vi "Opgave 9 Coolprop.vi"(10 "Temperatur":dbl, 11 "Tryk":dbl) -> (2 "Error Out":errorcluster, 3 "Entropy [kJ/kg-K]":dbl)   [LabVIEW 2019]
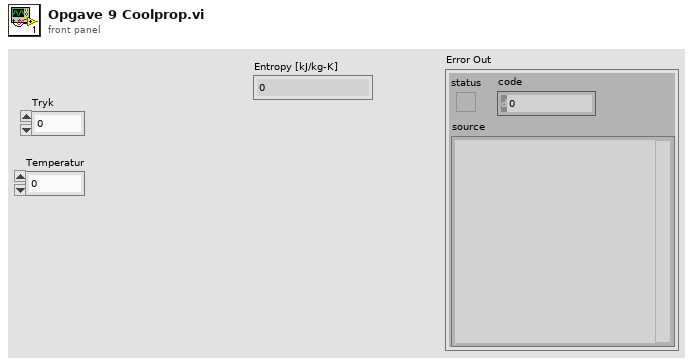
[diagram p1: front panel]
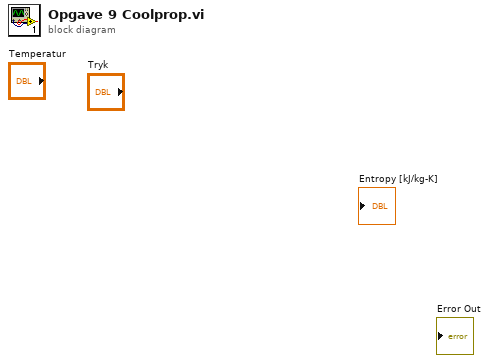
[diagram p0: block diagram]
diagram:
